vi "SYST_PRES.vi"(0 "VISA IN":refnum<visa-resource-name>, 5 "error in":errorcluster) -> (14 "VISA Out":refnum<visa-resource-name>, 19 "error out":errorcluster)   [LabVIEW 2018, in "PNA-X.lvlib"] (continued)
SCPI. \nParameters \n<cnum> Any existing channel number. If unspecified, value is set to 1 \n<char> Trigger mode. Choose from: \nHOLD - channel will not trigger \nCONTinuous - channel triggers indefinitely \nGROups - channel accepts the number of triggers specified with the last \nSENS:SWE:GRO:COUN <num>. This is one of the PNA overlapped commands. Learn \nmore. \nHow to specify Single Trigger - Internal or External: \n1. Send SENS:SWE:GRO:COUN 1 \n2. Send SENS:SWE:MODE GROups. When received, the specified PNA channel \nIMMEDIATELY accepts one trigger signal, if available, then goes into hold. To accept \nanother trigger signal, resend SENS:SWE:MODE GROups. \n1817\n\nExamples SENS:SWE:MODE CONT \nsense2:sweep:mode hold \nQuery Syntax SENSe<cnum>:SWEep:MODE? \nReturn Type Character \nDefault CONTinuous \nSENSe<cnum>:SWEep:POINts <num> \n(Read-Write) Sets the number of data points for the measurement. \nParameters \n<cnum> Any existing channel number. If unspecified, value is set to 1 \n<num> Choose any number between 1 and 16001 \nNote: This command will accept MIN or MAX instead of a numeric parameter. See SCPI \nSyntax for more information. \nExamples SENS:SWE:POIN 51 \nsense2:sweep:points max \nQuery Syntax SENSe<cnum>:SWEep:POINts? \nReturn Type Numeric \nDefault 201 \nSENSe<cnum>:SWEep:SRCPort <1 | 2> Superseded \nThis command is superseded. The Calc:Par:Def:Ext and Calc:Par:Mod:Ext can now optionally include the source \nport. \n(Read-Write) Sets the source port when making non S-parameter measurements. Has no effect on S-parameter \nmeasurements. \nParameters \n<cnum> Any existing channel number. If unspecified, value is set to 1 \n<1 | 2> 1 - Source power comes out Port 1 \n2 - Source power comes out Port 2 \nExamples SENS:SWE:SRCP 1 \nsense2:sweep:srcport 2 \nQuery Syntax SENSe<cnum>:SWEep:SRCPort? \n1818\n\nReturn Type Character \nDefault 1 \nSENSe<cnum>:SWEep:TIME <num> \n(Read-Write) Sets the time the analyzer takes to complete one sweep. If sweep time accuracy is critical, use \nONLY the values that are attained using the up and down arrows next to the sweep time entry box. See Sweep \nTime. \nParameters \n<cnum> Any existing channel number. If unspecified, value is set to 1 \n<num> Sweep time in seconds. Choose a number between 0 and 86,400 (24hrs), \nTo select the fastest sweep speed, either send MIN as an argument to this command, or \nsend SENS:SWE:TIME:AUTO 1 \nSee Note \nExamples SENS:SWE:TIME 1ms \nsense2:sweep:time .001 \nQuery Syntax SENSe<cnum>:SWEep:TIME? \nReturn Type Numeric \nDefault NA \nSENSe<cnum>:SWEep:TIME:AUTO <ON | OFF> \n(Read-Write) Turns the automatic sweep time function ON or OFF. \nParameters \n<cnum> Any existing channel number. If unspecified, value is set to 1 \n<ON | OFF> ON (or 1) - turns the automatic sweep time ON. \nOFF (or 0) - turns the automatic sweep time OFF. \nExamples SENS:SWE:TIME:AUTO \nsense2:sweep:time:auto off \nQuery Syntax SENSe<cnum>:SWEep:TIME:AUTO? \nReturn Type Boolean (1 = ON, 0 = OFF) \nDefault ON \n1819\n\nSENSe<cnum>:SWEep:TRIGger:DELay <num> \n(Read-Write) Sets and reads the trigger delay for all measurements in the specified CHANNEL. This delay is only \napplied while TRIG:SOURce EXTernal and TRIG:SCOP CURRent . After an external trigger is applied, the start \nof the sweep is delayed for the specified delay value plus any inherent latency. \nTo apply a trigger delay for all channels (Global), use TRIG:DEL \nParameters \n<cnum> Any existing channel number. If unspecified, value is set to 1 \n<num> Trigger delay value in seconds. Range is from 0 to 107 seconds \nExamples SENS:SWE:TRIG:DELay .003 \nsense2:sweep:trigger:delay 1 \nQuery Syntax SENSe<cnum>:SWEep:TRIGger:DELay? \nReturn Type Numeric \nDefault 0 \nSENSe<cnum>:SWEep:TRIGger:POINt <ON | OFF> \n(Read-Write) Specifies whether the specified channel will measure one point for each trigger or all of the \nmeasurements in the channel. Setting any channel to POINt mode will automatically set the TRIGger:SCOPe = \nCURRent.\nParameters \n<cnum> Any existing channel number. If unspecified, value is set to 1 \n<ON | OFF> ON (or 1) - Channel measures one data point per trigger. \nOFF (or 0) - All measurements in the channel made per trigger. \nExamples SENS:SWE:TRIG:POIN ON \nsense2:sweep:trigger:point off \nQuery Syntax SENSe<cnum>:SWEep:TRIGger:POINt? \nReturn Type Boolean (1 = Point, 0 = Measurement) \nDefault 0 - Measurement \nSENSe<cnum>:SWEep:TYPE <char> \n1820\n\n(Read-Write) Sets the type of analyzer sweep mode. \nParameters \n<cnum> Any existing channel number. If unspecified, value is set to 1 \n<char> Choose from: \nLINear | LOGarithmic | POWer | CW | SEGMent \nNote: SWEep TYPE cannot be set to SEGMent if there are no segments turned ON. A \nsegment is automatically turned ON when the analyzer is started. \nExamples SENS:SWE:TYPE LIN \nsense2:sweep:type segment \nQuery Syntax SENSe<cnum>:SWEep:TYPE? \nReturn Type Character \nDefault LINear \nLast Modified: \n24-Apr-2007 Clarified Sweep mode \n1821\n\nX Values Command \nSENSe<cnum>:X[:VALues]? \n(Read-only) Returns the stimulus values for the specified channel. If the channel is sweeping the \nsource backwards, the values will be in descending order. \nParameters \n<cnum> Any existing channel number; if unspecified, value is set to 1. \nExamples SENS:X? \nsense2:x:values? \nReturn Type Depends on FORM:DATA command \nDefault Not applicable \n1822\n\nSource Commands \nControls the power delivered to the DUT. \nClick on a blue keyword to view the command details. \nSee Also \nExample Programs \nLearn about Power Settings \nSynchronizing the PNA and Controller \nSCPI Command Tree \nSOURce<cnum>:CATalog? \n1823\n\n(Read-Write) Returns a list of valid port names that can be controlled. Some of these port names can \nNOT be accessed through the normal <port> argument used in many Source: commands. These string \nnames are used in the [src] argument. \nParameters \nExamples SOUR:CAT? \nsource:catalog \n'returns \n\"Port 1,Port 2,Port 3,Port 4,Port 1 Src2\" \nReturn Type Comma-separated list of strings. \nDefault Not applicable \nSOURce<cnum>:POWer<port>:ALC[:MODE]:CATalog?, [src] \n(Read-Write) Returns a list of valid ALC modes for the specified channel and port number. Use the \nreturned values to set SOUR:POW:ALC:MODE. \nParameters \n<cnum> Any existing channel number. If unspecified, value is set to 1 \n<port> Port number of the PNA. If unspecified, value is set to 1. To make settings for \nports that are not simple numbers, use the [src] argument. \n[src] String. (NOT case sensitive). Source port. Optional. Use SOUR:CAT? to \nreturn a list of valid port names. \nWhile this argument can be used to make settings for ALL ports, it is designed \nto access ports that are not simple numbers, such as \"Port 1 Src2\". Otherwise, \nthe <port> argument performs the same function. If both arguments are \nspecified, [src] takes priority. \nExamples SOUR:POW:ALC:MODE:CAT? \nsource2:power2:alc:mode:catalog? \nsource:power:alc:mode:catalog? \"Port 1 Src2\" \nReturn Type Comma-separated list of strings. \nDefault Not applicable \nSOURce<cnum>:POWer<port>:ALC[:MODE] <char>, [src] \n1824\n\n(Read-Write) Sets and returns the ALC mode for the specified channel and port. Use \nSOUR:POW:ALC:MODE:CAT? to return a list of valid ALC modes for the PNA. \nLearn more about ALC mode. \nParameters \n<cnum> Any existing channel number. If unspecified, value is set to 1 \n<port> Port number of the PNA. If unspecified, value is set to 1. To make settings for \nports that are not simple numbers, use the [src] argument. \n<char> ALC Mode. \nFor the PNA-X choose from: \nINTernal Standard ALC loop \nOPENloop No ALC loop \n[src] String. (NOT case sensitive). Source port. Optional. Use SOUR:CAT? to \nreturn a list of valid port names. \nWhile this argument can be used to make settings for ALL ports, it is designed \nto access ports that are not simple numbers, such as \"Port 1 Src2\". Otherwise, \nthe <port> argument performs the same function. If both arguments are \nspecified, [src] takes priority. \nExamples SOUR:POW:ALC INT \nsource2:power2:alc:mode openloop \nsource:power:alc:mode openloop,\"Port 1 Src2\" \nQuery Syntax SOURce<cnum>:POWer<port>:ALC:MODE? [src] \nReturn Type Character \nDefault INTernal \nSOURce<cnum>:POWer<port>:ATTenuation <num>, [src] \n1825\n\n(Read-Write) Sets the attenuation level for the selected channel. Sending this command turns \nautomatic attenuation control (SOUR:POW:ATT:AUTO) to OFF. If the ports are coupled, changing \nthe attenuation on one port will also change the attenuation on all other ports. To turn port coupling \nOFF use SOURce:POWer:COUPle OFF. \nNote: Attenuation cannot be set with Sweep Type set to Power \nParameters \n<cnum> Any existing channel number. If unspecified, value is set to 1 \n<port> Port number of the PNA. If unspecified, value is set to 1. To make settings for \nports that are not simple numbers, use the [src] argument. \n<num> Attenuation value. The range of settable values depends on the PNA model. \nTo determine the range of values, perform a query using MAX, then MIN, as \nan argument. Example: SOURce:POWer:ATT? Max \nEnter a value between MAX and MIN in 10 dB steps. \nIf a number other than these is entered, the analyzer will select the next lower \nvalid value. For example, if 19.9 is entered for <num> the analyzer will switch \nin 10 dB attenuation. \nNote: This command will accept MIN or MAX instead of a numeric \nparameter. See SCPI Syntax for more information. \n[src] String. (NOT case sensitive). Source port. Optional. Use SOUR:CAT? to \nreturn a list of valid port names. \nWhile this argument can be used to make settings for ALL ports, it is designed \nto access ports that are not simple numbers, such as \"Port 1 Src2\". Otherwise, \nthe <port> argument performs the same function. If both arguments are \nspecified, [src] takes priority. \nExamples SOUR:POW:ATT 10 \nsource2:power2:attentuation maximum \nsource:power:att 2, \"Port 1 Src2\" \nQuery Syntax SOURce<cnum>:POWer<port>:ATTenuation? [src] \nReturn Type Numeric \nDefault 0 \nSOURce<cnum>:POWer<port>:ATTenuation:AUTO <bool>, [src] \n1826\n\n(Read-Write) Turns automatic attenuation control ON or OFF. Setting an attenuation value (using \nSOURce:POWer:ATTenuation <num>) sets AUTO OFF. \nParameters \n<cnum> Any existing channel number. If unspecified, value is set to 1. \n<port> Port number of the PNA. If unspecified, value is set to 1.To make settings for \nports that are not simple numbers, use the [src] argument. \n<bool> ON (or 1) - turns coupling ON. The analyzer automatically selects the \nappropriate attenuation level to meet the specified power level. \nOFF (or 0) - turns coupling OFF. Attenuation level must be set using \nSOURce:POWer:ATTenuation <num>. \n[src] String. (NOT case sensitive). Source port. Optional. Use SOUR:CAT? to \nreturn a list of valid port names. \nWhile this argument can be used to make settings for ALL ports, it is designed \nto access ports that are not simple numbers, such as \"Port 1 Src2\". Otherwise, \nthe <port> argument performs the same function. If both arguments are \nspecified, [src] takes priority. \nExamples SOUR:POW2:ATT:Auto On \nsource2:power:attentuation:auto off \nsour:pow:att:auto 1, \"Port 1 Src2\" \nQuery Syntax SOURce<cnum>:POWer:ATTenuation:Auto? [src] \nReturn Type Boolean (1 = ON, 0 = OFF) \nDefault ON \nSOURce<cnum>:POWer:CENTer <num> \n1827\n\n(Read-Write) Sets the power sweep center power. Must also set: \nSENS:SWE:TYPE POWer and SOURce:POWer:SPAN <num>. \nParameters \n<cnum> Any existing channel number. If unspecified, value is set to 1 \n<num> Center power. Actual achievable leveled power depends on frequency. \nExamples SOUR:POW:CENT -15 \nsource2:power:center -7 \nQuery Syntax SOURce<cnum>:POWer:CENTer? \nReturn Type Numeric \nDefault 0 dBm \nSOURce<cnum>:POWer:COUPle <ON | OFF> \n(Read-Write) Turns Port Power Coupling ON or OFF. \nParameters \n<cnum> Any existing channel number. If unspecified, value is set to 1 \n<ON | OFF> ON (or 1) - turns coupling ON. The same power level is used for both source \nports. \nOFF (or 0) - turns coupling OFF. Power level can be set individually for each \nsource port. \nExamples SOUR:POW:COUP ON \nsource2:power:couple off \nQuery Syntax SOURce<cnum>:POWer:COUPle? \nReturn Type Boolean (1 = ON, 0 = OFF) \nDefault ON \nSOURce<cnum>:POWer:DETector <char> OBSOLETE \n1828\n\n(Read-Write) The PNA models with external leveling are now OBSOLETE. \nSets the source leveling loop as Internal or External. \nParameters \n<cnum> Any existing channel number. If unspecified, value is set to 1 \n<char> INTernal - Internal leveling is applied to the source \nEXTernal - External leveling is applied to the source through a rear-panel \nconnector. ONLY provided on 3 GHz, 6 GHz, and 9 GHz PNA models. \nExamples SOUR:POW:DET INT \nsource2:power:detector external \nQuery Syntax SOURce<cnum>:POWer:DETector? \nReturn Type Character \nDefault INTernal \nSOURce<cnum>:POWer<port>[:LEVel][:IMMediate] \n[:AMPLitude] <num>, [src] \n(Read-Write) Sets the RF power output level. \nParameters \n<cnum> Any existing channel number. If unspecified, value is set to 1 \n<port> Port number of the PNA. If unspecified, value is set to 1. To make settings for \nports that are not simple numbers, use the [src] argument. \n<num> Source power in dBm. \nNote: The range of settable power values depends on the PNA model and if \nsource attenuators are installed. To determine the range of values, perform a \nquery using MAX, then MIN, as an argument. (SOUR:POW:ATT:AUTO must \nbe set to ON) Example: SOURce:POWer? Max \nActual achievable leveled power depends on frequency. \n[src] String. (NOT case sensitive). Source port. Optional. Use SOUR:CAT? to \nreturn a list of valid port names. \nWhile this argument can be used to make settings for ALL ports, it is designed \nto access ports that are not simple numbers, such as \"Port 1 Src2\". Otherwise, \nthe <port> argument performs the same function. If both arguments are \nspecified, [src] takes priority.\n1829\n\nExamples SOUR:POW1 5DB \nsource2:power:level:immediate:amplitude maximum \nsour:pow 5, \"Port 1 Src2\" \nQuery Syntax SOURce<cnum>:POWer[:LEVel][:IMMediate][:AMPLitude]? [src] \nReturn Type Numeric \nDefault 0 dBm \nSOURce<cnum>:POWer[:LEVel]:SLOPe <num> \n(Read-Write) Sets the RF power slope value. \nParameters \n<cnum> Any existing channel number. If unspecified, value is set to 1 \n<num> Slope value in db/GHz. Choose any integer between -2 and 2 (0 is no slope). \nExamples SOUR:POW:SLOP 2 \nsource2:power:slope -2 \nQuery Syntax SOURce<cnum>:POWer[:LEVel]:SLOPe? \nReturn Type Numeric \nDefault 0 \nSOURce<cnum>:POWer[:LEVel]:SLOPe:STATe <ON | OFF> \n(Read-Write) Turns Power Slope ON or OFF. \nParameters \n<cnum> Any existing channel number. If unspecified, value is set to 1 \n<ON|OFF> ON (or 1) - turns slope ON. \nOFF (or 0) - turns slope OFF. \nExamples SOUR:POW:SLOP:STAT ON \nsource2:power:slope:state off \nQuery Syntax SOURce<cnum>:POWer[:LEVel]:SLOPe:STATe? \nReturn Type Boolean (1 = ON, 0 = OFF) \nDefault OFF \nSOURce<cnum>:POWer<port>:MODE <state>, [src] \n1830\n\n(Read-Write) Sets the state of PNA source for the specified port. \nLearn more about the PNA internal second source \nParameters \n<cnum> Any existing channel number. If unspecified, value is set to 1 \n<port> Port number of the PNA. If unspecified, <port> is set to 1. To make settings for \nports that are not simple numbers, use the [src] argument. \n<state> Source state. Choose from: \nAUTO Source power is turned ON when required for a measurement. \nON Source power is always ON regardless of the measurement. \nOFF Source power is always OFF regardless of the measurement. \nNote: ON and OFF are valid only on PNA models with two sources. \n[src] String. (NOT case sensitive). Source port. Optional. Use SOUR:CAT? to \nreturn a list of valid port names. \nWhile this argument can be used to make settings for ALL ports, it is designed \nto access ports that are not simple numbers, such as \"Port 1 Src2\". Otherwise, \nthe <port> argument performs the same function. If both arguments are \nspecified, [src] takes priority. \nExamples SOUR:POW:MODE ON \nsource2:power4:mode OFF \nsour:pow:mode 1, \"Port 1 Src2\" \nQuery Syntax SOURce<cnum>:POWer<port>:MODE? [src} \nReturn Type Character \nDefault Auto \nSOURce<cnum>:POWer:SPAN <num> \n1831\n\n(Read-Write) Sets the power sweep span power. Must also set: \nSENS:SWE:TYPE POWer and SOURce:POWer:CENTer <num>. \nParameters \n<cnum> Any existing channel number. If unspecified, value is set to 1. \n<num> Span power. Actual achievable leveled power depends on frequency. \nExamples SOUR:POW:SPAN -15 \nsource2:power:span -7 \nQuery Syntax SOURce<cnum>:POWer:SPAN? \nReturn Type Numeric \nDefault 0 dBm \nSOURce<cnum>:POWer:STARt <num> \n(Read-Write) Sets the power sweep start power. Must also set \nSENS:SWE:TYPE POWer and SOURce:POWer:STOP <num>. \nParameters \n<cnum> Any existing channel number. If unspecified, value is set to 1 \n<num> Start power. \nNote: The range of settable power values depends on the PNA model and if \nsource attenuators are installed. To determine the range of values, perform a \nquery using MAX, then MIN, as an argument. (SOUR:POW:ATT:AUTO must \nbe set to ON) Example: SOURce:POWer:STARt? MIN \nActual achievable leveled power depends on frequency. \nExamples SOUR:POW:STAR -15 \nsource2:power:start -7 \nQuery Syntax SOURce<cnum>:POWer:STARt? \nReturn Type Numeric \nDefault 0 dBm \nSOURce<cnum>:POWer:STOP <num> \n1832\n\n(Read-Write) Sets the power sweep stop power. Must also set: SENS:SWE:TYPE POWer and \nSOURce:POWer:START <num>. \nParameters \n<cnum> Any existing channel number. If unspecified, value is set to 1 \n<num> Stop power. \nNote: The range of settable power values depends on the PNA model and if \nsource attenuators are installed. To determine the range of values, perform a \nquery using MAX, then MIN, as an argument. (SOUR:POW:ATT:AUTO must \nbe set to ON) Example: SOURce:POWer:STOP? MAX \nActual achievable leveled power depends on frequency. \nExamples SOUR:POW:STOP -15 \nsource2:power:stop -7 \nQuery Syntax SOURce<cnum>:POWer:STOP? \nReturn Type Numeric \nDefault 0 dBm \nLast modified: \n10/18/06 MQQ Added Mode command \n1833\n\nSource:Power:Correction Commands \nControls the source power calibration features of the analyzer. \nClick on a blue keyword to view the command details. \nSee Also \nExample program using these commands. \nTemplate for creating your own Power Meter Driver \nLearn about Source Power Cal \nSynchronizing the PNA and Controller \nSCPI Command Tree \nNote: The SOURce:POWer:CORRection:COLLect:ACQuire command, used to step the PNA and read a \npower meter, cannot be sent over the GPIB unless the power meter is connected to a different GPIB \ninterface. See the alternative methods described in the command details. \nSOURce<cnum>:POWer<port>:CORRection:COLLect:ABORt \n1834\n\n(Write-only) Aborts a source power calibration sweep that is in progress. \nParameters \n<cnum> Any existing channel number. If unspecified, value is set to 1 \n<port> Port number to correct for source power. If unspecified, value is set to 1. \nExamples SOUR:POW:CORR:COLL:ABOR \nsource1:power2:correction:collect:abort \nQuery Syntax Not Applicable \nDefault Not Applicable \nSOURce<cnum>:POWer<port>:CORRection:COLLect[:ACQuire] <char>,<id>[,src] \nNote: With PNA Rev. 6.2, a new \"id\" argument has been added to this command, replacing \nSOUR:POW:CORR:COLL:METH. \n(Write-only) Initiates a source power cal acquisition sweep using the power sensor attached to the \nspecified channel (A or B) on the power meter, or using the specified PNA receiver. \nNote: This command, when used with a power meter, cannot be sent over the GPIB unless the power \nmeter is connected to a different GPIB interface. Use one of the following methods to perform this \ncommand or its equivalent: \nIf present, use the GPIB dedicated controller port. \nConnect the power meter to the PNA using a USB / GPIB interface (Agilent 82357A). \nSCPI programming of the PNA using a LAN Client interface (see example) \nSend SCPI commands through the COM interface using the SCPI String Parser object. \nDirectly control the Power Meter and PNA to step frequency; then acquire and store the Power reading. \n(see example). \nParameters \n<cnum> Any existing channel number. If unspecified, value is set to 1 \n<port> Port number to correct for source power. If unspecified, value is set to 1. \n<char> The following choices are new beginning PNA Rev 6.2. Choose from: \nPMETer - Power Meter is used for all readings. \nPMReceiver - Power meter for the first iteration; then use the reference receiver \nfor remaining readings if necessary (same as \"fast iteration\" box checked on \n1835\n\ndialog box) \nRECeiver - Use PNA measurement receiver for all readings. \nThe following choices are superseded but still supported, in conjunction with \nSOUR:POW:CORR:COLL:METH. \nASENsor - Sensor on power meter channel A \nBSENsor - Sensor on power meter channel B \n<id> String. Not case sensitive. The power sensor or PNA receiver to use for \nmeasuring power. \nFor PMETer or PMRECeiver: select \"ASENSOR\" or \"BSENSOR\". \nFor RECeiver: select a PNA receiver to acquire readings using physical or logical \nreceiver notation. \nFor ASENsor or BSENsor, this argument is NOT required. \n[src] String. (NOT case sensitive). Source port. Optional. Use SOUR:CAT? to \nreturn a list of valid port names. \nWhile this argument can be used to make settings for ALL ports, it is designed \nto access ports that are not simple numbers, such as \"Port 1 Src2\". Otherwise, \nthe <port> argument performs the same function. If both arguments are \nspecified, [src] takes priority. \nExamples SOUR:POW:CORR:COLL PMET 'acquires power meter readings using \nthe A sensor. \nsource1:power2:correction:collect:acquire receiver,\"a1\" \n'acquires source cal readings using the reference receiver for \nport 1. \nQuery Syntax Not Applicable \nDefault Not Applicable \nSOURce:POWer:CORRection:COLLect:AVERage[:COUNt] <num> \n1836\n\n(Read-Write) This command, along with SOUR:POW:CORR:COLL:AVER:NTOLerance, allows for \nsettling of the power sensor READINGS. \nSpecifies the maximum number of power readings that are taken at each stimulus point to allow for \nmeasurement settling. Each reading is averaged with the previous readings at that stimulus point. \nWhen this average meets the Average:NTOLerance value or this number of readings has been made, \nthe average is returned as the valid reading. \nThis setting is not necessary when using a PNA receiver (SOUR:POW:CORR:COLL REC) to make \nthe measurement. \nLearn more. \nParameters \n<num> Maximum number of readings to make to allow for settling. Choose any \nnumber between 3 and 25. \nExamples SOUR:POW:CORR:COLL:AVER 2 \nsource:power:correction:collect:average:count 3 \nQuery Syntax SOURce:POWer:CORRection:COLLect:AVERage[:COUNt]? \nReturn Type Numeric \nDefault 3 \nSOURce:POWer:CORRection:COLLect:AVERage:NTOLerance <num> \n(Read-Write) This command, along with SOUR:POW:CORR:COLL:AVER:COUNT, allows for \nsettling of the power sensor READINGS. \nEach power reading is averaged with the previous readings at each stimulus point. When the average \nmeets this nominal tolerance value or the max number of readings has been made, the average is \nreturned as the valid reading. \nThis setting is not necessary when using a PNA receiver (SOUR:POW:CORR:COLL REC) to make \nthe measurement. \nLearn more. \nParameters \n<num> Power measurement settling tolerance value in dB. Choose any number \nbetween 0 and 5. \nExamples SOUR:POW:CORR:COLL:AVER:NTOL .05 \nsource1:power2:correction:collect:average:ntolerance .003 \n1837\n\nQuery Syntax SOURce:POWer:CORRection:COLLect:AVERage:NTOLerance? \nReturn Type Numeric \nDefault .050 dBm \nSOURce<cnum>:POWer:CORRection:COLLect:DISPlay[:STATe] <ON | OFF> \n(Read-Write) Enables and disables the display of power readings on the PNA screen. Send this \ncommand BEFORE you begin a source power cal acquisition. After the source power cal data is \nacquired, this setting is reset to ON. \nParameters \n<cnum> Any existing channel number. If unspecified, value is set to 1 \n<ON|OFF> ON (1) Source power calibration dialog box is shown on the PNA screen. \nPower readings are plotted against the Tolerance value as limit lines. \nOFF (0) - Source power calibration dialog box is NOT shown on the PNA \nscreen. \nExamples SOUR:POW:CORR:COLL:DISP ON \nsource1:power2:correction:collect:display:state off \nQuery Syntax SOURce:POWer:CORRection:COLLect:DISPlay[:STATe]? \nReturn Type Boolean (1 = ON, 0 = OFF) \nDefault ON (1) \nSOURce<cnum>:POWer:CORRection:COLLect:FCHeck[:STATe] <ON | OFF> \n(Read-Write) Enables and disables frequency checking of source power cal acquisition sweeps. \nONLY use when you have more than one power sensor. \nParameters \n<cnum> Any existing channel number. If unspecified, value is set to 1 \n<ON|OFF> ON (1) turns source power cal frequency checking ON. A requested \nacquisition will only succeed for those frequency points which fall within a \nfrequency range specified for the power sensor being used. An acquisition will \npause in mid-sweep if the frequency is about to exceed the maximum \nfrequency limit specified for that sensor. When the sweep is paused in this \nmanner, a sensor connected to the other channel input of the power meter can \nbe connected to the measurement port in place of the previous sensor, and used \nto complete the sweep. However, the maximum frequency specified for the \n1838\n\nsecond sensor would need to be sufficient for the sweep to complete. \nFrequency limits are specified using the SOUR:POW:CORR:COLL:SEN \ncommand. \nOFF (0) - turns source power cal frequency checking OFF. An acquisition will \nuse just one power sensor for the entire sweep, regardless of frequency. \nExamples SOUR:POW:CORR:COLL:FCH ON \nsource1:power2:correction:collect:fcheck:state off \nQuery Syntax SOURce:POWer:CORRection:COLLect:FCHeck[:STATe]? \nReturn Type Boolean (1 = ON, 0 = OFF) \nDefault OFF (0) \nSOURce:POWer:CORRection:COLLect:ITERation[:COUNt] <num> \n(Read-Write) This command, along with SOUR:POW:CORR:COLL:ITER:NTOL describes the \nnumber of ADUSTMENTS to make to the source power. \nSets the maximum number of readings to take at each data point for iterating the source power. Power \nREADINGS (performed by SOUR:POW:CORR:COLL:AVER:COUNT and \nSOUR:POW:CORR:COLL:AVER:NTOLerance) will continue to be made, and source power \nadjusted, until the measurement is within the iteration tolerance value or this max number of \nmeasurements has been met. The last value is the valid measurement for that data point. \nLearn more. \nParameters \n<num> Maximum number of readings. Choose any number between 1 and 100. \nExamples SOUR:POW:CORR:COLL:ITER 2 \nsource:power:correction:collect:iteration 3 \nQuery Syntax SOURce:POWer:CORRection:COLLect:ITERation[:COUNt]? \nReturn Type Numeric \nDefault 1 \nSOURce:POWer:CORRection:COLLect:ITERation:NTOLerance <num> \n1839\n\n(Read-Write) This command, along with SOUR:POW:CORR:COLL:ITER:COUNT describes the \nnumber of ADUSTMENTS to make to the source power. \nSets the maximum desired deviation from the sum of the test port power and the offset value. Power \nREADINGS (performed by SOUR:POW:CORR:COLL:AVER:COUNT and \nSOUR:POW:CORR:COLL:AVER:NTOLerance) will continue to be made, and source power \nadjusted, until a measurement is within this tolerance value or the max number of measurements has \nbeen met. The last value is the valid measurement for that data point. \nLearn more. \nParameters \n<cnum> Any existing channel number. If unspecified, value is set to 1 \n<port> Port number to correct for source power. If unspecified, value is set to 1. \n<num> Tolerance value in dBm. Choose any number between 0 and 5 \nExamples SOUR:POW:CORR:COLL:ITER:NTOL .005 \nsource:power:correction:collect:iteration:ntolerance .1 \nQuery Syntax SOURce:POWer:CORRection:COLLect:ITERation:NTOLerance? \nReturn Type Numeric \nDefault .05 \nSOURce<cnum>:POWer<port>:CORRection:COLLect:METHod <char> Superseded \nThis command is replaced with SOUR:POW:CORR:COLLect[:ACQuire] which now specifies the \nmethod and the device. \n(Read-Write) Selects the calibration method to be used for the source power cal acquisition. \nParameters \n<cnum> Any existing channel number. If unspecified, value is set to 1 \n<port> Port number to correct for source power. If unspecified, value is set to 1. \n<char> Choose from: \nNONE - No Cal method \nPMETer - Power Meter is used for all readings. (same as \"fast iteration\" box \nnot checked on dialog box) \nPMReceiver - Power meter for the first iteration; then use the reference \nreceiver for remaining readings if necessary (same as \"fast iteration\" box \n1840\n\nchecked on dialog box) \nExamples SOUR:POW:CORR:COLL:METH PMET \nsource1:power2:correction:collect:method pmreceiver \nQuery Syntax SOURce:POWer:CORRection:COLLect:METHod? \nReturn Type Character \nDefault NONE \nSOURce<cnum>:POWer<port>:CORRection:COLLect:SAVE [<RREC>] \n(Write-only) Applies the array of correction values after a source power calibration sweep has \ncompleted. The source power correction will then be active on the specified source port for channel \n<cnum>. This command does NOT save the correction values. To save correction values, save an \ninstrument / calibration state (*.cst file) after performing a source power cal. \nParameters \n<cnum> Any existing channel number. If unspecified, value is set to 1 \n<port> Port number to correct for source power. If unspecified, value is set to 1. \n<RREC> Optional argument. \nRRECeiver In addition to a source Power Cal, perform a calibration of the \nreference receiver used in the measurement. ONLY the Reference Receiver \ncalibration is then saved to a Cal Set or Cal Register as specified by the current \nsetting of SENS:CORR:PREF:CSET:SAVE. \nExamples SOUR:POW:CORR:COLL:SAVE \nsource1:power2:correction:collect:save rreceiver \nQuery Syntax Not Applicable \nDefault Not Applicable \nSOURce<cnum>:POWer:CORRection:COLLect:<pmChan>SENsor[:FRANge] \n<num1>,<num2> \n1841\n\n(Read-Write) Specifies the frequency range over which the power sensors connected to the specified \nchannels (A and B) of the power meter can be used (minimum frequency, maximum frequency). If the \npower meter has only a single channel, that channel is considered channel A. \nParameters \n<cnum> Any existing channel number. If unspecified, value is set to 1 \n<pmChan> Power Meter channel. Choose from: \nA - Channel A \nB - Channel B \n<num1> Minimum frequency for the sensor. If a frequency unit is not specified, Hz is \nassumed. No limits are placed on this value. \n<num2> Maximum frequency for the sensor. If a frequency unit is not specified, Hz is \nassumed. No limits are placed on this value. \nExamples SOUR:POW:CORR:COLL:ASEN 100E3, 3E9 \nsource1:power2:correction:collect:bsensor:frange 10 MHz, 18 GHz \nQuery Syntax SOURce:POWer:CORRection:COLLect:ASENsor[:FRANge]? \nSOURce:POWer:CORRection:COLLect:BSENsor[:FRANge]? \nReturn Type Numeric \nDefault 0,0 \nSOURce<cnum>:POWer:CORRection:COLLect:<pmChan>SENsor:RCFactor <num> \n(Read-Write) ) Specifies the reference cal factor for the power sensor connected to channel A or B of \nthe power meter. If the power meter has only a single channel, that channel is considered channel A. \nNote: If the sensor connected to the specified channel of the power meter contains cal factors in \nEPROM (such as the Agilent E-series power sensors), those will be the cal factors used during the \ncalibration sweep. The reference cal factor value associated with this command, and any cal factors \nentered into the PNA for that sensor channel, will not be used. \nParameters \n<cnum> Any existing channel number. If unspecified, value is set to 1 \n<pmChan> Power Meter channel. Choose from: \nA - Channel A \nB - Channel B \n1842\n\n<num> Reference cal factor in percent. Choose any number between 1 and 150. \nExamples SOUR:POW:CORR:COLL:ASEN:RCF 98.7 \nsource1:power2:correction:collect:bsensor:rcfactor 105 \nQuery Syntax SOURce:POWer:CORRection:COLLect:ASENsor:RCFactor? \nSOURce:POWer:CORRection:COLLect:BSENsor:RCFactor? \nReturn Type Numeric \nDefault 100 \nSOURce<cnum>:POWer:CORRection:COLLect:<pmChan>SENsor:SELect \n(Read-Write) Sets and returns the power sensor channel (A or B) to be used. This performs the same \nfunction as the Use this sensor only checkbox in the Power Sensor Settings dialog. \nNote: This write portion of this command is only necessary when performing an SMC calibration. \nParameters \n<cnum> Any existing channel number. If unspecified, value is set to 1 \n<pmChan> Power Meter channel. Choose from: \nA - Channel A \nB - Channel B \nExamples SOUR:POW:CORR:COLL:<pmChan>SEN:SEL 'Write \nsource1:power2:correction:collect:bsensor:select? 1e9 'Read \nQuery Syntax SOURce:POWer:CORRection:COLLect:ASENsor:SELect? <Frequency> \nSOURce:POWer:CORRection:COLLect:BSENsor:SELect? <Frequency> \nReturns a boolean 1 or 0 (true or false) indicating whether the sensor is to be \nused at the specified frequency. \nIf frequency checking is OFF, then the <Frequency> parameter is ignored. The \nquery returns if the sensor is selected for ALL frequencies. \nReturn Type Numeric \nDefault Not Applicable \nSOURce<cnum>:POWer:CORRection:COLLect:TABLe:DATA <data> \n1843\n\n(Read-Write) Read or write data into the selected table. Use \nSOUR:POW:CORR:COLL:TABL:SELect to select a table. \nIf the selected table is a power sensor table, the data is interpreted as cal factors in percent. \nIf the loss table is selected, the data is interpreted as loss in dB. \nParameters \n<cnum> Any existing channel number. If unspecified, value is set to 1 \n<data> Data to write into the selected table. \nExamples SOURce:POWer:CORRection:COLLect:TABLe:DATA 0.12, 0.34, 0.56 \nQuery Syntax SOURce<cnum>:POWer:CORRection:COLLect:TABLe:DATA? \nIf the selected table is currently empty, no data is returned. \nReturn Type Numeric - one number per table segment. \nDefault Not Applicable \nSOURce<cnum>:POWer:CORRection:COLLect:TABLe:FREQuency <data> \n(Read-Write) Read or write frequency values for the selected table (cal factor table for a power sensor, \nor the loss compensation table). \nParameters \n<cnum> Any existing channel number. If unspecified, value is set to 1 \n<data> Frequency data to write into the selected table. \nExamples SOURce:POWer:CORRection:COLLect:TABLe:FREQuency 10E6, 1.5E9, 9E9 \nQuery Syntax SOURce<cnum>:POWer:CORRection:COLLect:TABLe:FREQuency? \nIf the selected table is currently empty, no data is returned. \nReturn Type Numeric - one number per table segment \nDefault Not Applicable \nSOURce<cnum>:POWer:CORRection:COLLect:TABLe:LOSS[:STATe] <ON | OFF> \n1844\n\n(Read-Write) Indicates whether or not to adjust the power readings using the values in the loss table \nduring a source power cal sweep. \nParameters \n<cnum> Any existing channel number. If unspecified, value is set to 1 \n<ON|OFF> ON (or 1) - turns use of the loss table ON. \nOFF (or 0) - turns use of the loss table OFF. \nExamples SOUR:POW:CORR:COLL:TABL:LOSS ON \nsource1:power2:correction:collect:table:loss:state off \nQuery Syntax SOURce:POWer:CORRection:COLLect:TABLe:LOSS[:STATe]? \nReturn Type Boolean (1 = ON, 0 = OFF) \nDefault OFF (0) \nSOURce<cnum>:POWer:CORRection:COLLect:TABLe:POINts? \n(Read-only) Returns the number of segments that are currently in the selected table. \nParameters \n<cnum> Any existing channel number. If unspecified, value is set to 1 \nExamples SOUR:POW:CORR:COLL:TABL:POIN? \nsource1:power2:correction:collect:table:points? \nReturn Type Numeric \nDefault 0 \nSOURce<cnum>:POWer:CORRection:COLLect:TABLe[:SELect] <char> \n1845\n\n(Read-Write) Selects which table you want to write to or read from. Read or write using \nSOURce:POWer:CORRection:COLLect:TABLe:FREQuency and \nSOURce:POWer:CORRection:COLLect:TABLe:DATA \nParameters \n<cnum> Any existing channel number. If unspecified, value is set to 1 \n<char> Choose from: \nNONE - No table selected \nASENsor - Cal Factor table for Power Sensor A \nBSENsor - Cal Factor table for Power Sensor B \nLOSS - Loss compensation table \nExamples SOUR:POW:CORR:COLL:TABL ASEN \nsource1:power2:correction:collect:table:select bsensor \nQuery Syntax SOURce:POWer:CORRection:COLLect:TABLe[:SELect]? \nReturn Type Character \nDefault NONE \nSOURce<cnum>:POWer<port>:CORRection:DATA <data>[,src] \n(Read-Write) Writes and reads source power calibration data. \nWhen querying source power calibration data, if no source power cal data exists for the specified \nchannel and source port, then no data is returned. \nIf a change in the instrument state causes interpolation and/or extrapolation of the source power cal, \nthe correction data associated with this command correspond to the new instrument state (interpolated \nand/or extrapolated data). \nIf the channel is sweeping the source backwards, then the first data point is the highest frequency \nvalue; the last data point is the lowest. Use the SENS:X:VALues? command to return the X-axis \nvalues in the displayed order. \nParameters \n<cnum> Any existing channel number. If unspecified, value is set to 1 \n<port> Port number to correct for source power. If unspecified, value is set to 1. \n<data> Correction Data \n1846\n\n[src] String. (NOT case sensitive). Source port. Optional. Use SOUR:CAT? to \nreturn a list of valid port names. \nWhile this argument can be used to make settings for ALL ports, it is designed \nto access ports that are not simple numbers, such as \"Port 1 Src2\". Otherwise, \nthe <port> argument performs the same function. If both arguments are \nspecified, [src] takes priority. \nExamples SOURce1:POWer2:CORRection:DATA 0.12, -0.34, 0.56 \nQuery Syntax SOURce<cnum>:POWer<port>:CORRection:DATA? [src] \nReturn Type Depends on FORMat:DATA command \nDefault Not Applicable \nSOURce<cnum>:POWer<port>:CORRection:LEVel <num>[,src] \n(Read-Write) Specifies the power level that is expected at the desired reference plane (DUT input or \noutput). This is not used for segment sweep with independent power levels or power sweeps. \nNote: Although this command still works, it is recommended that you specify cal power by setting the \ntest port power and offset value. \nParameters \n<cnum> Any existing channel number. If unspecified, value is set to 1 \n<port> Port number to correct for source power. If unspecified, value is set to 1. \n<num> Cal power level in dBm. Because this could potentially be at the output of a \ndevice-under-test, no limits are placed on this value here. It is realistically \nlimited by the specifications of the device (power sensor) that will be used for \nmeasuring the power. The power delivered to the PNA receiver must never \nexceed PNA specifications for the receiver! \n[src] String. (NOT case sensitive). Source port. Optional. Use SOUR:CAT? to \nreturn a list of valid port names. \nWhile this argument can be used to make settings for ALL ports, it is designed \nto access ports that are not simple numbers, such as \"Port 1 Src2\". Otherwise, \nthe <port> argument performs the same function. If both arguments are \nspecified, [src] takes priority. \nExamples SOUR:POW:CORR:LEV 10 \nsource1:power2:correction:level 0 dbm \nQuery Syntax SOURce:POWer:CORRection:LEVel? [src] \n1847\n\nReturn Type Numeric \nDefault 0 dBm \nSOURce<cnum>:POWer<port>:CORRection:OFFSet[:MAGNitude] <num>[,src] \n(Read-Write) Sets or returns a power level offset from the PNA test port power. This can be a gain or \nloss value (in dB) to account for components you connect between the source and the reference plane \nof your measurement. For example, specify 10 dB to account for a 10 dB amplifier at the input of your \nDUT. \nCal power is the sum of the test port power setting and this offset value. Following the calibration, the \nPNA power readouts are adjusted to the cal power. \nParameters \n<cnum> Any existing channel number. If unspecified, value is set to 1 \n<port> Port number to correct for source power. If unspecified, value is set to 1. \n<num> Gain or loss value in dB. Choose a value between -200 and 200 \n[src] String. (NOT case sensitive). Source port. Optional. Use SOUR:CAT? to \nreturn a list of valid port names. \nWhile this argument can be used to make settings for ALL ports, it is designed \nto access ports that are not simple numbers, such as \"Port 1 Src2\". Otherwise, \nthe <port> argument performs the same function. If both arguments are \nspecified, [src] takes priority. \nExamples SOUR:POW:CORR:OFFS 10 \nsource1:power2:correction:offset:magnitude -3 \nQuery Syntax SOURce:POWer:CORRection:OFFSet[:MAGNitude]? [src] \nReturn Type Numeric \nDefault 0 dB \nSOURce<cnum>:POWer<port>:CORRection[:STATe] <bool>[,src] \n1848\n\n(Read-Write) Enables and disables source power correction for the specified port on the specified \nchannel. \nParameters \n<cnum> Any existing channel number. If unspecified, value is set to 1 \n<port> Port number to correct for source power. If unspecified, value is set to 1. \n<bool> ON (or 1) turns source power correction ON. \nOFF (or 0) - turns source power correction OFF. \n[src] String. (NOT case sensitive). Source port. Optional. Use SOUR:CAT? to return a list \nof valid port names. \nWhile this argument can be used to make settings for ALL ports, it is designed to \naccess ports that are not simple numbers, such as \"Port 1 Src2\". Otherwise, the <port> \nargument performs the same function. If both arguments are specified, [src] takes \npriority. \nExamples SOUR:POW:CORR ON \nsource1:power2:correction:state off \nQuery \nSyntax \nSOURce:POWer:CORRection[:STATe]? [src] \nReturn \nType \nBoolean (1 = ON, 0 = OFF) \nDefault OFF (0) \nLast modified: \nApril 17, 2007 Removed ch and port arguments for 4 settling and accuracy commands. \n9/12/06 MQ Modified for receiver only SPC \n1849\n\nStatus Register Commands \nThe status registers enable you to query the state of selected events that occur in the analyzer. \nNote: This documentation requires familiarity with the \"Standard Status Data Structure - Register \nModel\" as defined in IEEE Std 488.2-1992. \nClick on a blue keyword to view the command details. \nSee Also \nExample Programs \nLearn about Status Registers \nSynchronizing the PNA and Controller \nSCPI Command Tree \nNote: Any bit not shown in the registers is not used but may be reserved for future use. \n1850\n\nStatus Byte Register \nSummarizes the states of the other registers and monitors the PNA output queue. It also generates \nservice requests. The Enable register is called the Service Request Enable Register. \nCommands Description \n*CLS Clears ALL \"event\" registers and the SCPI Error / Event queue. The corresponding \nENABLE registers are unaffected. \n*STB? Reads the value of the analyzer's status byte. The byte remains after being read. \n*SRE? Reads the current state of the Service Request Enable Register. \n*SRE <num> Sets bits in the Service Request Enable register. The current setting of the SRE \nregister is stored in non-volatile memory. Use *SRE 0 to clear the enable. \n<num> Combined value of the weights for bits to be set. \nBit Weight Description Bit is set to 1 when the following conditions exist: \n2 4 Error / Event \nqueue Summary \n(EAV) \nthe Error / Event queue is not empty. To read the error \nmessage, use SYST:ERR? \n3 8 Questionable \nRegister Summary \nany enabled bit in the questionable event status register is \nset to 1 \n4 16 Message Available the output queue is not empty \n5 32 Standard Event \nRegister Summary \nany enabled bit in the standard event status register is set to \n1 \n6 64 Request Service any of the other bits in the status byte register is set to 1 \n(used to alert the controller of a service request within the \nanalyzer). This bit cannot be disabled. \n7 128 Operation Register \nSummary \nany enabled bit in the standard operation event status \nregister is set to 1 \n1851\n\nSTATus:QUEStionable:<keyword> \nSummarizes conditions that monitor the quality of measurement data. \n<keyword> Example \n:CONDition? STAT:QUES:COND? \n:ENABle \n<bits> \nSTAT:QUES:ENAB 1024 \n[:EVENt]? STAT:QUES? \n:NTRansition \n<bits> \nSTAT:QUES:NTR 1024 \n:PTRansition \n<bits> \nSTAT:QUES:PTR 0 \nBit Weight Description Bit is set to 1 when the following conditions exist: \n9 512 Integrity Reg \nsummary \nany enabled bit in the Integrity event register is set to 1 \n10 1024 Limit Registers \nsummary \nany enabled bit in the Limit event registers is set to 1 \n11 2048 Define Registers \nsummary \nany enabled bit in the Define event registers is set to 1 \nSTATus:QUEStionable:INTegrity <keyword> \nSummarizes conditions in the Measurement Integrity register. \n<keyword> Example \n:CONDition? STAT:QUES:INT:COND? \n:ENABle <bits> STAT:QUES:INT:ENAB 1024 \n[:EVENt]? STAT:QUES:INT? \n:NTRansition <bits> STAT:QUES:INT:NTR 1024 \n:PTRansition <bits> STAT:QUES:INT:PTR 0 \n1852\n\nBit Weight Description Bit is set to 1 when the following conditions exist: \n0 1 Measurement \nSummary \nany bit in the Measurement Integrity event register is set to \n1 \n2 4 Hardware \nSummary \nany bit in the Hardware event register is set to 1 \nSTATus:QUEStionable:INTegrity:HARDware<keyword> \nMonitors the status of hardware failures. \n<keyword> Example \n:CONDition? STAT:QUES:INT:HARD:COND? \n:ENABle <bits> STAT:QUES:INT:HARD:ENAB 1024 \n[:EVENt]? STAT:QUES:INT:HARD? \n:NTRansition <bits> STAT:QUES:INT:HARD:NTR 1024 \n:PTRansition <bits> STAT:QUES:INT:HARD:PTR 0 \nBit Weight Description Bit is set to 1 when the following conditions exist: \n1 2 Phase Unlock the source has lost phaselock, possibly caused by a reference \nchannel open or a hardware failure. \n2 4 Unleveled the source power is unleveled. This could be caused by a \nsource set for more power than it can deliver at the tuned \nfrequency. Or it could be caused by a hardware failure. \n3 8 Not used N/A \n4 16 EE Write Failed an attempted write to the EEPROM has failed, possibly \ncaused by a hardware failure. \n5 32 Not used N/A \n6 64 Ramp Cal Failed the analyzer was unable to calibrate the analog ramp \ngenerator due to a possible hardware failure. \n7 128 Not used N/A \n1853\n\nSTATus:QUEStionable:INTegrity:MEASurement<n> <keyword> \nMonitors the lag between changing a channel setting and when the data is ready to query. \nWhen you change the channel state (start/stop freq, bandwidth, and so forth), then the questionable bit \nfor that channel is set. This indicates that your desired channel state does not yet match the data you \nwould get if querying a data trace. When the next sweep is complete (without aborting in the middle), \nand the data trace matches the channel state that produced it, the bit is cleared for that channel. \n<n> Measurement register number. Choose from 1 to 3 \n<keyword> Example \n:CONDition? STAT:QUES:INT:MEAS1:COND? \n:ENABle <bits> STAT:QUES:INT:MEAS2:ENAB 1024 \n[:EVENt]? STAT:QUES:INT:MEAS3? \n:NTRansition <bits> STAT:QUES:INT:MEAS2:NTR 1024 \n:PTRansition <bits> STAT:QUES:INT:MEAS1:PTR 0 \nMeasurement Register <n> \nBit Weight 1 2 3 Bit is set to 1 when the following conditions exist: \n0 1 1 Summary \nfrom \nMeas \nReg 3 \na setting change on this channel has occurred and the \ndata does not yet reflect that change. \n1 2 2 15 29 a setting change on this channel has occurred and the \ndata does not yet reflect that change. \n2 4 3 16 30 a setting change on this channel has occurred and the \ndata does not yet reflect that change. \n3 8 4 17 31 a setting change on this channel has occurred and the \ndata does not yet reflect that change. \n4 16 5 18 32 a setting change on this channel has occurred and the \ndata does not yet reflect that change. \n5 32 6 19 a setting change on this channel has occurred and the \ndata does not yet reflect that change. \n6 64 7 20 a setting change on this channel has occurred and the \ndata does not yet reflect that change. \n1854\n\n7 128 8 21 a setting change on this channel has occurred and the \ndata does not yet reflect that change. \n8 256 9 22 a setting change on this channel has occurred and the \ndata does not yet reflect that change. \n9 512 10 23 a setting change on this channel has occurred and the \ndata does not yet reflect that change. \n10 1024 11 24 a setting change on this channel has occurred and the \ndata does not yet reflect that change. \n11 2048 12 25 a setting change on this channel has occurred and the \ndata does not yet reflect that change. \n12 4096 13 26 a setting change on this channel has occurred and the \ndata does not yet reflect that change. \n13 8192 14 27 a setting change on this channel has occurred and the \ndata does not yet reflect that change. \n14 16384 Summary \nfrom \nMeas \nReg 2 \n28 a setting change on this channel has occurred and the \ndata does not yet reflect that change. \nSTATus:QUEStionable:LIMit<n> <keyword> \nMonitors and summarizes the status of limit line failures. When a trace fails, the representative bit is \nset to 1. \nBit 0 is used to summarize failures in the registers that follow. For example, Limit Register 3, bit 0, \nsummarizes the failures from registers 4 through 10. \nAll enable bits are set to 1 by default. \nTo find the measurement number, use Calc:Par:Mnum \n<n> Limit register: Choose from 1 to 10. \n<keyword> Example \n:CONDition? STAT:QUES:LIM4:COND? \n:ENABle <bits> STAT:QUES:LIM1:ENAB 1024 \n[:EVENt]? STAT:QUES:LIM3? \n:NTRansition <bits> STAT:QUES:LIM2:NTR 1024 \n:NTRansition? STAT:QUES:LIM1:NTR? \n1855\n\n:PTRansition <bits> STAT:QUES:LIM5:PTR 0 \n:PTRansition? STAT:QUES:LIM1:PTR? \nLimit Register <n> \nBit Weight 1 2 3 4 5 6 7 8 ... 41 Bit is set to 1 when the \nfollowing conditions exist: \n0 1 2-42 3-42 4-42 5-42 6-42 7-42 8-42 9-42 ... 42 Summary Bit - If any bit \nfrom that register fails, it \npropagates to the previous \nregister, bit 0. \nTrace Numbers \n1 2 1 15 29 43 57 71 85 99 ... 575 any point on trace fails the \nlimit test \n2 4 2 16 30 44 58 72 86 100 ... 576 any point on trace fails the \nlimit test \n3 8 3 17 31 45 59 73 87 101 ... 577 any point on trace fails the \nlimit test \n4 16 4 18 32 46 60 74 88 102 ... 578 any point on trace fails the \nlimit test \n5 32 5 19 33 47 61 75 89 103 ... 579 any point on trace fails the \nlimit test \n6 64 6 20 34 48 62 76 90 104 ... 580 any point on trace fails the \nlimit test \n7 128 7 21 35 49 63 77 91 105 ... -- any point on trace fails the \nlimit test \n8 256 8 22 36 50 64 78 92 106 ... -- any point on trace fails the \nlimit test \n9 512 9 23 37 51 65 79 93 107 ... -- any point on trace fails the \nlimit test \n10 1024 10 24 38 52 66 80 94 108 ... -- any point on trace fails the \nlimit test \n11 2048 11 25 39 53 67 81 95 109 ... -- any point on trace fails the \nlimit test \n1856\n\n12 4096 12 26 40 54 68 82 96 110 ... -- any point on trace fails the \nlimit test \n13 8192 13 27 41 55 69 83 97 111 ... -- any point on trace fails the \nlimit test \n14 16384 14 28 42 56 70 84 98 112 ... -- any point on trace fails the \nlimit test \nTo determine Register, Bit number, and Weight for trace numbers between 113 and 574 (not shown in \nthe above table) use the following calculations. \nThe limit status for trace numbers higher than 580 can NOT be tracked. \nThe following example calculates the Register, Bit number, and Bit Weight for trace # 400: \nTo determine Limit Register number, use ((Trace # - 1) / 14) + 1. \nTo determine Limit Bit Number, use the remainder +1 of the above calculation. \n((400-1)/14) + 1 = Register# r+1Bit \n399/14 = 28 r7 \n28+1= Register 29 \n7+1= Bit number 8 \nTo determine Limit Bit Weight: Use above table. For example: Bit 8 = 256 \nSTATus:QUEStionable:DEFine<keyword> \nSummarizes conditions in the Questionable:Define:User<1|2|3> event registers. \n<keyword> Example \n:CONDition? STAT:QUES:DEF:COND? \n:ENABle <bits> STAT:QUES:DEF:ENAB 1024 \n[:EVENt]? STAT:QUES:DEF? \n:NTRansition <bits> STAT:QUES:DEF:NTR 1024 \n:PTRansition <bits> STAT:QUES:DEF:PTR 0 \n1857\n\nBit Weight Description Bit is set to 1 when the following conditions exist: \n1 2 USER1 any bit in the USER1 event register is set to 1 \n2 4 USER2 any bit in the USER2 event register is set to 1 \n3 8 USER3 any bit in the USER3 event register is set to 1 \nSTATus:QUEStionable:DEFine:USER<1|2|3><keyword> \nMonitors conditions that you define and map in any of the three QUES:DEF:USER event registers. \n<keyword> Example \n:ENABle <bits> STAT:QUES:DEF:USER1:ENABle 1024 \n[:EVENt]? STAT:QUES:DEF:USER1? \n:MAP <bit>,<error> STAT:QUES:DEF:USER1:MAP 0,-113 'when error -113 occurs, \nbit 0 in USER1 will set to 1. \nBit Weight Description Bit is set to 1 when the following conditions exist: \n0 1 for user user defined \n1 2 for user user defined \n2 4 for user user defined \n3 8 for user user defined \n4 16 for user user defined \n5 32 for user user defined \n6 64 for user user defined \n7 128 for user user defined \n8 256 for user user defined \n9 512 for user user defined \n10 1024 for user user defined \n11 2048 for user user defined \n12 4096 for user user defined \n13 8192 for user user defined \n14 16384 for user user defined \n1858\n\nStandard Event Status Register \nMonitors \"standard\" events that occur in the analyzer. This register can only be cleared by: \na Clear Command (*CLS). \nreading the Standard Enable Status Register (*ESE?). \na power-on transition. The analyzer clears the register and then records any transitions that occur, including \nsetting the Power On bit (7). \nCommands Description \n*ESE? Reads the settings of the standard event ENABLE register. \n*ESE <bits> Sets bits in the standard event ENABLE register. The current setting is saved in \nnon-volatile memory. \n<bits> The sum of weighted bits in the register. Use *ESE 0 to clear the enable \nregister. \n*ESR? Reads and clears the EVENT settings in the Standard Event Status register. \n*OPC Sets bit 0 when the overlapped command is complete. (see Understanding \nCommand Synchronization / OPC). \n*OPC? Operation complete query - read the Operation Complete bit (0). \nBit Weight Description Bit is set to 1 when the following conditions exist: \n0 1 Operation \nComplete \nthe two following events occur in order: \nthe *OPC command is sent to the analyzer 1. \nthe analyzer completes all pending overlapped commands 2. \n1 NA Request \nControl \nNot Supported - the analyzer application is not configured to \ncontrol GPIB operation \n2 4 Query Error a query error is detected indicating: \n- an attempt to read data from the output queue when no data was \npresent OR \n- data in the output queue was lost, as in an overflow \n4 16 Execution \nError \nan execution error is detected indicating: \n- a <PROGRAM DATA> element was outside the legal range or \ninconsistent with the operation of the analyzer OR \n1859\n\n- the analyzer could not execute a valid command due to some \ninternal condition \n5 32 Command \nError \na command error is detected indicating that the analyzer received \na command that: \ndid not follow proper syntax \nwas misspelled \nwas an optional command it does not implement \n7 128 Power ON Power to the analyzer has been turned OFF and then ON since the \nlast time this register was read. \nSTATus:OPERation<keyword> \nSummarizes conditions in the Averaging and Operation:Define:User<1|2|3> event registers. \n<keyword> Example \n:CONDition? STAT:OPER:COND? \n:ENABle <bits> STAT:OPER:ENAB 1024 \n[:EVENt]? STAT:OPER? \n:NTRansition <bits> STAT:OPER:NTR 1024 \n:PTRansition <bits> STAT:OPER:PTR 0 \nBit Weight Description Bit is set to 1 when the following conditions exist: \n8 256 Averaging \nsummary \neither enabled bit in the Averaging summary event register is set \nto 1 \n9 512 User Defined \nsummary \n10 1024 Device \nsummary \neither enabled bit in the Device summary event register is set to \n1 \n1860\n\nSTATus:OPERation:AVERaging<n> <keyword> \nMonitors and summarizes the status of Averaging on traces 1 to 128. When averaging for a trace is \ncomplete, the representative bit is set to 1. \nBit 0 is used to summarize the status in the registers that follow. For example, Average Register, bit 0, \nsummarizes the status from registers 4 through 10. \nAll enable bits are set to 1 by default. \nTo find the measurement number, use Calc:Par:Mnum. \n<n> Averaging Register. Choose from 1 to 10 \n<keyword> Example \n:CONDition? STAT:OPER:AVER1:COND? \n:ENABle <bits> STAT:OPER:AVER1:ENAB 1024 \n[:EVENt]? STAT:OPER:AVER1? \n:NTRansition <bits> STAT:OPER:AVER1:NTR 1024 \n:PTRansition <bits> STAT:OPER:AVER1:PTR 0 \nAveraging Register <n> \nBit Weight 1 2 3 4 5 6 7 8 ... 42 Bit is set to 1 when the \nfollowing conditions exist: \n0 1 2-42 3-42 4-42 5-42 6-42 7-42 8-42 9-42 ... 42 Summary Bit - If any bit \nfrom that register fails, it \npropagates to the previous \nregister, bit 0. \nTrace Numbers \n1 2 1 15 29 43 57 71 85 99 ... 575 Averaging on this trace is \ncomplete \n2 4 2 16 30 44 58 72 86 100 ... 576 Averaging on this trace is \ncomplete \n3 8 3 17 31 45 59 73 87 101 ... 577 Averaging on this trace is \ncomplete \n4 16 4 18 32 46 60 74 88 102 ... 578 Averaging on this trace is \ncomplete \n1861\n\n5 32 5 19 33 47 61 75 89 103 ... 579 Averaging on this trace is \ncomplete \n6 64 6 20 34 48 62 76 90 104 ... 580 Averaging on this trace is \ncomplete \n7 128 7 21 35 49 63 77 91 105 ... -- Averaging on this trace is \ncomplete \n8 256 8 22 36 50 64 78 92 106 ... -- Averaging on this trace is \ncomplete \n9 512 9 23 37 51 65 79 93 107 ... -- Averaging on this trace is \ncomplete \n10 1024 10 24 38 52 66 80 94 108 ... -- Averaging on this trace is \ncomplete \n11 2048 11 25 39 53 67 81 95 109 ... -- Averaging on this trace is \ncomplete \n12 4096 12 26 40 54 68 82 96 110 ... -- Averaging on this trace is \ncomplete \n13 8192 13 27 41 55 69 83 97 111 ... -- Averaging on this trace is \ncomplete \n14 16384 14 28 42 56 70 84 98 112 ... -- Averaging on this trace is \ncomplete \nTo determine Register, Bit number, and Weight for trace numbers between 113 and 574 (not shown in \nthe above table) use the following calculations. \nThe averaging status for trace numbers higher than 580 can NOT be tracked. \nThe following example calculates the Register, Bit number, and Bit Weight for trace # 400: \nTo determine Register number, use ((Trace # - 1) / 14) + 1. \nTo determine Bit Number, use the remainder +1 of the above calculation. \n((400-1)/14) + 1 = Register# r+1Bit \n399/14 = 28 r7 \n28+1= Register 29 \n7+1= Bit number 8 \n1862\n\nTo determine Bit Weight: Use above table. For example: Bit 8 = 256 \nSTATus:OPERation:DEFine<keyword> \nSummarizes conditions in the OPERation:Define:User<1|2|3> event registers. \n<keyword> Example \n:CONDition? STAT:OPER:DEF:COND? \n:ENABle <bits> STAT:OPER:DEF:ENAB 12 \n[:EVENt]? STAT:OPER:DEF? \n:NTRansition <bits> STAT:OPER:DEF:NTR 12 \n:PTRansition <bits> STAT:OPER:DEF:PTR 0 \nBit Weight Description Bit is set to 1 when the following conditions exist: \n1 2 USER1 any bit in the USER1 event register is set to 1 \n2 4 USER2 any bit in the USER2 event register is set to 1 \n3 8 USER3 any bit in the USER3 event register is set to 1 \nSTATus:OPERation:DEFine:USER<1|2|3><keyword> \nMonitors conditions that you define and map in any of the three OPER:DEF:USER event registers. \n<keyword> Example \n:ENABle <bits> STAT:OPER:DEF:USER1:ENAB 1024 \n[:EVENt]? STAT:OPER:DEF:USER1? \n:MAP <bit>,<error> STAT:OPER:DEF:USER1:MAP 0,-113 'when error -113 occurs, \nbit 0 in USER1 will set to 1. \n1863\n\nBit Weight Description Bit is set to 1 when the following conditions exist: \n0 1 for user user defined \n1 2 for user user defined \n2 4 for user user defined \n3 8 for user user defined \n4 16 for user user defined \n5 32 for user user defined \n6 64 for user user defined \n7 128 for user user defined \n8 256 for user user defined \n9 512 for user user defined \n10 1024 for user user defined \n11 2048 for user user defined \n12 4096 for user user defined \n13 8192 for user user defined \n14 16384 for user user defined \nSTATus:OPERation:DEVice<keyword> \nSummarizes conditions in the OPERation:DEVice event registers. \n<keyword> Example \n:CONDition? STAT:OPER:DEV:COND? \n:ENABle <bits> STAT:OPER:DEV:ENAB 16 \n[:EVENt]? STAT:OPER:DEV? \n:NTRansition <bits> STAT:OPER:DEV:NTR 16 \n:PTRansition <bits> STAT:OPER:DEV:PTR 0 \n1864\n\nBit Weight Description Bit is set to 1 when the following conditions exist: \n0 1 Unused \n1 2 Unused \n2 4 Unused \n3 8 Unused \n4 16 Sweep Completed When sweep is complete \n5 32 Unused \n6 64 Unused \n7 128 Unused \n8 256 Unused \n9 512 Unused \n10 1024 Unused \n11 2048 Unused \n12 4096 Unused \n13 8192 Unused \n14 16384 Unused \nLast modified: \nMay 31, 2007 Fixed typo in STAT:QUES:INT register \n9/19/06 MQ Modified for unlimited windows. \n1865\n\nSystem Commands \n1866\n\n1867\n\nClick on a blue keyword to view the command details. \nSee Also \nExample Programs \nLearn about Preset \nSynchronizing the PNA and Controller \nSCPI Command Tree"
uses:
  PNA-X.lvlib
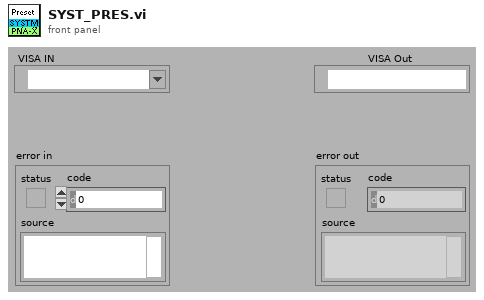
[diagram p1: front panel]
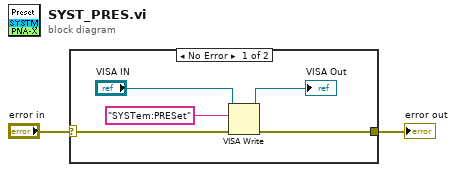
[diagram p0: block diagram]
diagram:
  n1 = case shown="No Error" "error in" {
    selector: "error in" -> [w3 w8]
    tunnel: [w6 w8] -> w1
    frame No Error {
      n2 = VISA Write(VISA resource name="VISA IN", write buffer="SYSTem:PRESet" ("Cmdline"), error in (no error)=w3) -> (VISA resource name out=→"VISA Out":refnum<visa-resource-name>, error out=w6:errorcluster)  [unwired: 1 out]
    }
    frame Error {
    }
  }
  "error out" <- w1
